vi "FIFO_AUTO_TEST.vi"() -> ()   [LabVIEW 2023]
uses:
  <vilib>/numeric/Random Number (Range) I64.vi
  deps/hdl-shared/host_interfaces/fifo/LabVIEW/HdlFifo/NiFpga_HdlFifo_WriteI64.vi
  deps/hdl-shared/host_interfaces/fifo/LabVIEW/HdlFifo/NiFpga_HdlFifo_ReadI64.vi
  <vilib>/numeric/Random Number (Range) DBL.vi
  deps/hdl-shared/host_interfaces/fifo/LabVIEW/HdlFifo/NiFpga_HdlFifo_WriteSGL.vi
  deps/hdl-shared/host_interfaces/fifo/LabVIEW/HdlFifo/NiFpga_HdlFifo_ReadSGL.vi
  <vilib>/numeric/Random Number (Range) U64.vi
  deps/hdl-shared/host_interfaces/fifo/LabVIEW/HdlFifo/NiFpga_HdlFifo_WriteU64.vi
  deps/hdl-shared/host_interfaces/fifo/LabVIEW/HdlFifo/NiFpga_HdlFifo_ReadU64.vi
  deps/hdl-shared/host_interfaces/fifo/LabVIEW/HdlFifo/NiFpga_HdlFifo_WriteBool.vi
  deps/hdl-shared/host_interfaces/fifo/LabVIEW/HdlFifo/NiFpga_HdlFifo_ReadBool.vi
  deps/hdl-shared/host_interfaces/fifo/LabVIEW/HdlFifo/NiFpga_HdlFifo_WriteI8.vi
  deps/hdl-shared/host_interfaces/fifo/LabVIEW/HdlFifo/NiFpga_HdlFifo_ReadI8.vi
  deps/hdl-shared/host_interfaces/fifo/LabVIEW/HdlFifo/NiFpga_HdlFifo_WriteU16.vi
  deps/hdl-shared/host_interfaces/fifo/LabVIEW/HdlFifo/NiFpga_HdlFifo_ReadU16.vi
  deps/hdl-shared/host_interfaces/fifo/LabVIEW/HdlFifo/NiFpga_HdlFifo_WriteI32.vi
  deps/hdl-shared/host_interfaces/fifo/LabVIEW/HdlFifo/NiFpga_HdlFifo_ReadI32.vi
  <vilib>/numeric/sub_Random U32.vi
  <vilib>/FPGAPlugInAG/Dynamic/niLvFpga_Download_Dynamic.vi
  <vilib>/FPGAPlugInAG/Dynamic/niLvFpga_Run_Dynamic.vi
  deps/hdl-shared/host_interfaces/fifo/LabVIEW/HdlFifo/NiFpga_HdlFifo_AddI64.vi
  deps/hdl-shared/host_interfaces/fifo/LabVIEW/HdlFifo/private/_NiFpga_HdlFifo_GetStream.vi
  <vilib>/Utility/error.llb/Error Cluster From Error Code.vi
  deps/hdl-shared/host_interfaces/fifo/LabVIEW/HdlFifo/NiFpga_HdlFifo_AddSGL.vi
  deps/hdl-shared/host_interfaces/fifo/LabVIEW/HdlFifo/NiFpga_HdlFifo_AddU64.vi
  deps/hdl-shared/host_interfaces/fifo/LabVIEW/HdlFifo/NiFpga_HdlFifo_AddBool.vi
  deps/hdl-shared/host_interfaces/fifo/LabVIEW/HdlFifo/NiFpga_HdlFifo_AddI8.vi
  deps/hdl-shared/host_interfaces/fifo/LabVIEW/HdlFifo/NiFpga_HdlFifo_AddU16.vi
  deps/hdl-shared/host_interfaces/fifo/LabVIEW/HdlFifo/NiFpga_HdlFifo_AddI32.vi
  <vilib>/rvi/interface/nirviMethod/nirviMethod.xnode
panel:
  in  "Access non-existant FIFOs":bool
  out "error out 8":errorcluster
  out "Non-Existant FIFO test status":bool
  in  "I64 Multiplier 2":sgl
  out "Numeric 9":i32
  in  "SGL Multiplier":dbl
  in  "U64 Multiplier":sgl
  in  "I8 Multiplier":sgl
  in  "U16 Multiplier":sgl
  in  "I32 Multiplier":sgl
  in  "I64 Multiplier":sgl
  out "error out 7":errorcluster
  out "I64 Pass":bool
  out "Numeric 8":i32
  out "WriteData 6":i64[](array[numeric])
  out "ReadData 6":i64[](array[numeric])
  in  "Device address":string="PXI1Slot2"
  in  "Bitfile path":path=path "C:/shared/github15-test/MacallanTop_GH15_7dmatest_3.lvbitx"
  out "data out":bool[](array[boolean])
  out "Array":bool[](array[boolean])
  out "Numeric 2":i32
  out "Boolean Pass":bool
  out "Numeric 7":i32
  out "WriteData 5":u64[](array[numeric])
  out "ReadData 5":u64[](array[numeric])
  out "U64 Pass":bool
  out "Numeric 6":i32
  out "WriteData 4":sgl[](array[numeric])
  out "ReadData 4":sgl[](array[numeric])
  out "SGL Pass":bool
  out "error out 6":errorcluster
  out "error out 5":errorcluster
  out "error out 4":errorcluster
  out "error out 3":errorcluster
  out "error out 2":errorcluster
  out "error out":errorcluster
  out "Numeric 5":i32
  out "WriteData 3":i8[](array[numeric])
  out "ReadData 3":i8[](array[numeric])
  out "I8 Pass":bool
  out "Numeric 4":i32
  out "WriteData 2":u16[](array[numeric])
  out "ReadData 2":u16[](array[numeric])
  out "U16 Pass":bool
  out "ReadData":i32[](array[numeric])
  out "WriteData":i32[](array[numeric])
  out "Numeric":i32
  out "I32 Pass":bool
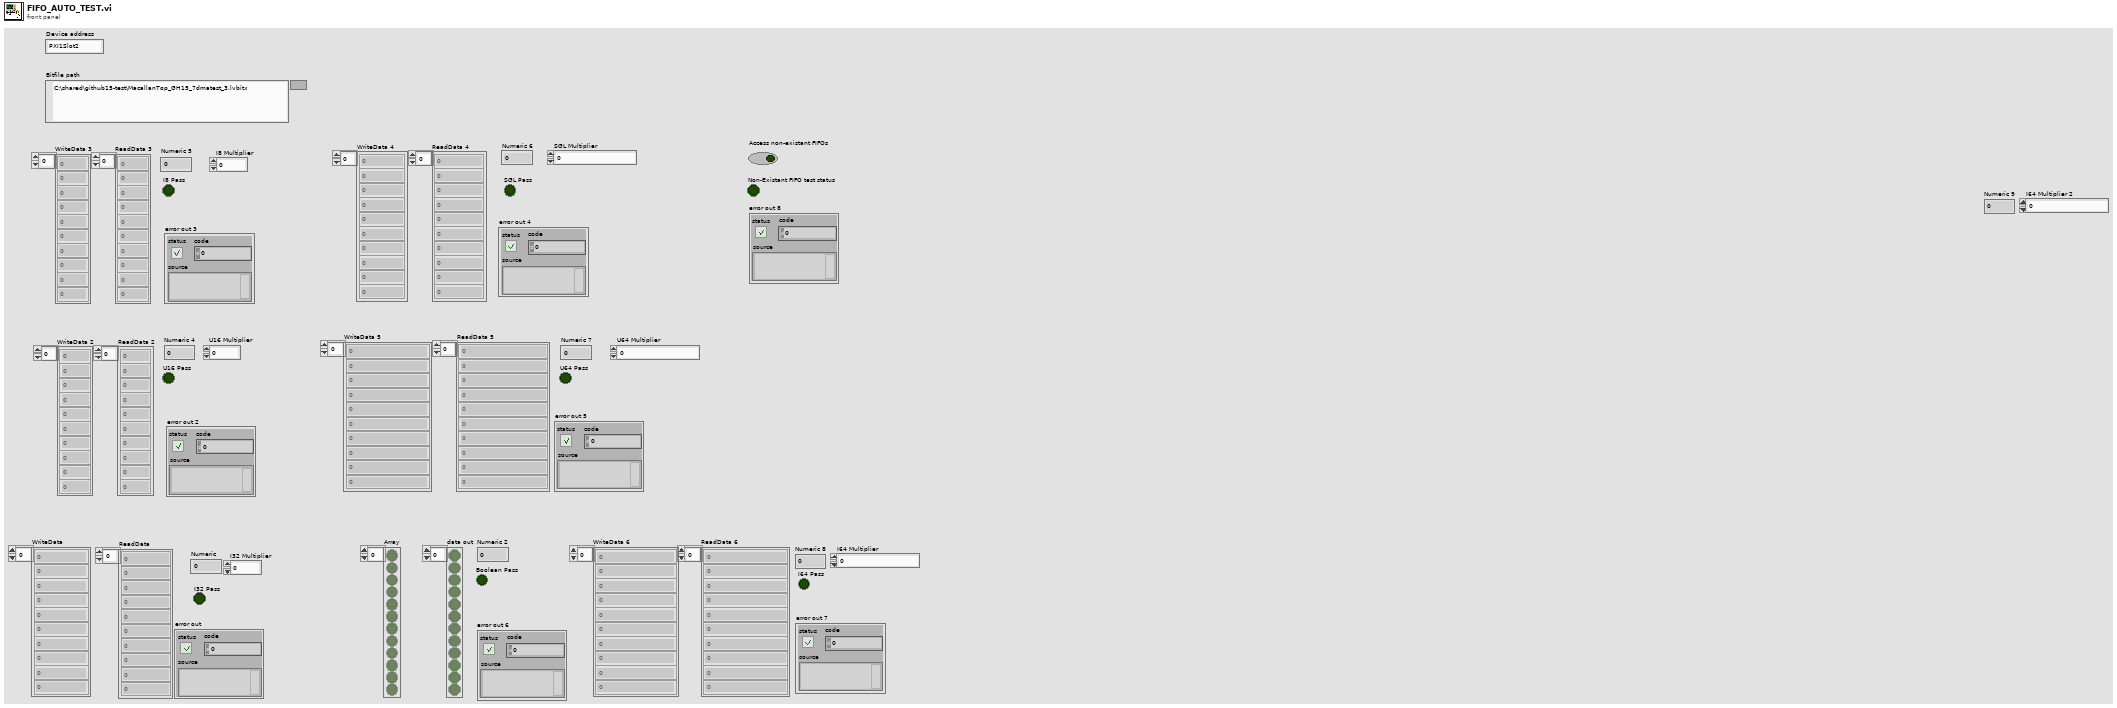
[diagram p1: front panel]
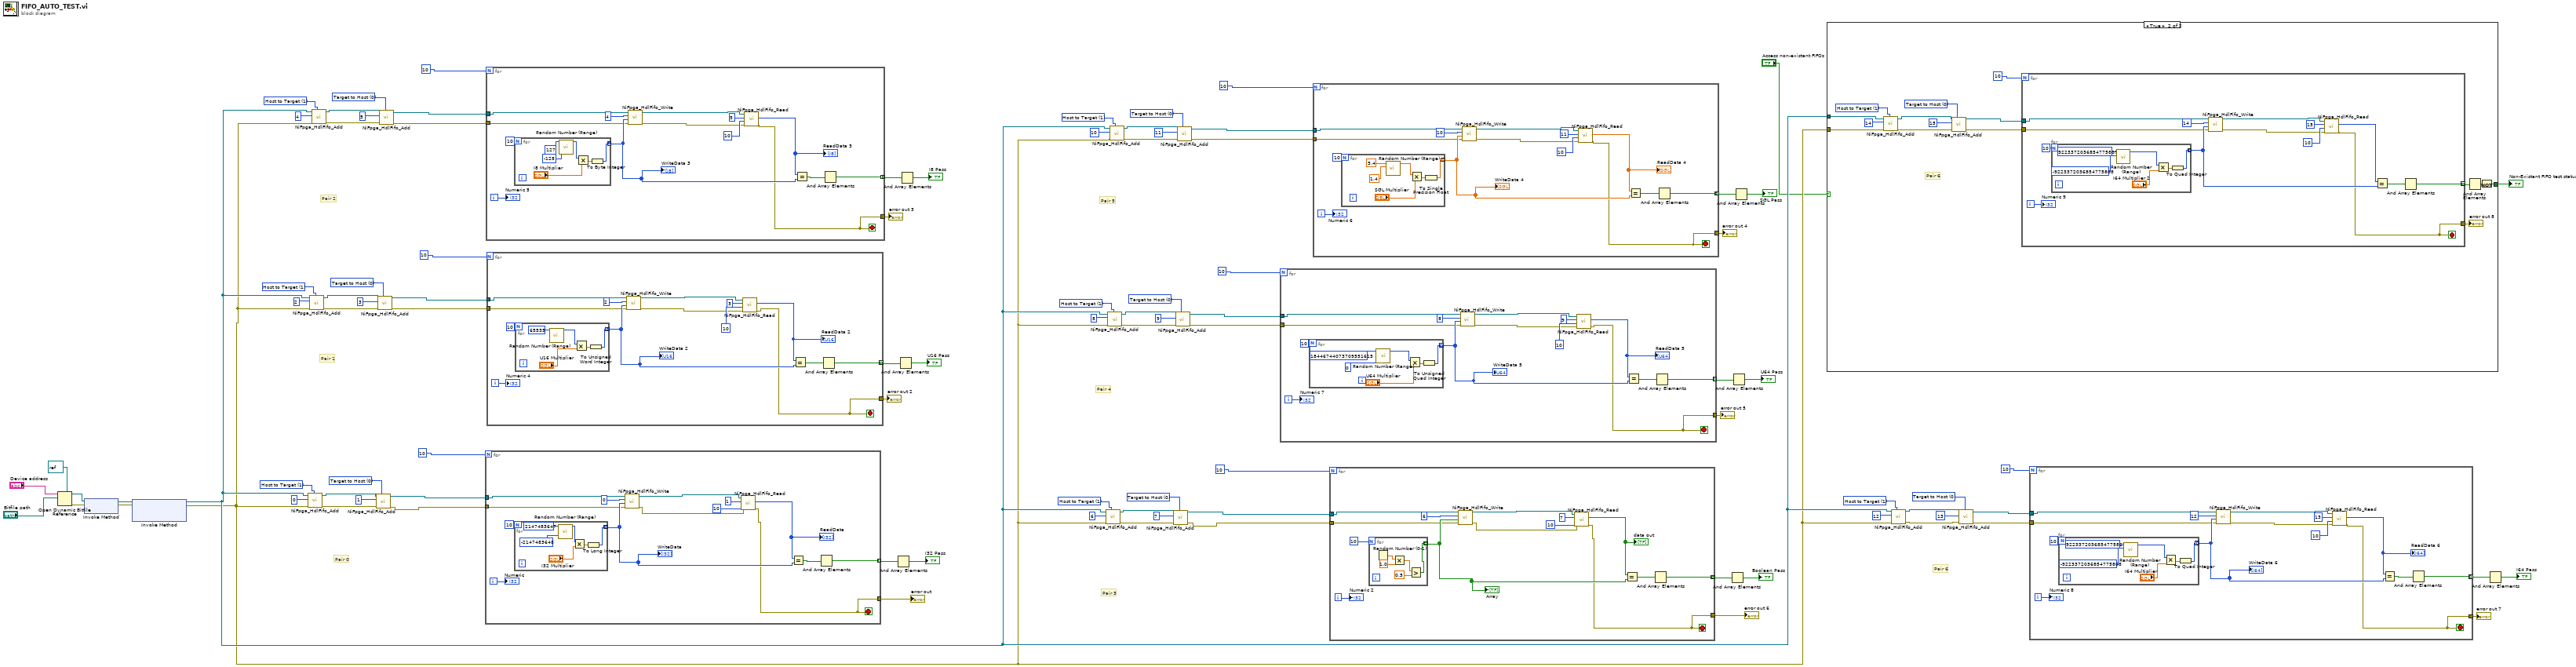
[diagram p0: block diagram]
diagram:
  w10 = u32 0 items=["Target to Host", "Host to Target"] ("direction")
  w6 = u32 1 items=["Target to Host", "Host to Target"]
  w39 = u32 0 items=["Target to Host", "Host to Target"] ("direction")
  w35 = u32 1 items=["Target to Host", "Host to Target"]
  w30 = u32 0 items=["Target to Host", "Host to Target"] ("direction")
  w34 = u32 1 items=["Target to Host", "Host to Target"]
  w21 = u32 0 items=["Target to Host", "Host to Target"] ("direction")
  w17 = u32 1 items=["Target to Host", "Host to Target"]
  w66 = u32 0 items=["Target to Host", "Host to Target"] ("direction")
  w70 = u32 1 items=["Target to Host", "Host to Target"]
  w75 = u32 0 items=["Target to Host", "Host to Target"] ("direction")
  w71 = u32 1 items=["Target to Host", "Host to Target"]
  w85 = u32 0 items=["Target to Host", "Host to Target"] ("direction")
  w89 = u32 1 items=["Target to Host", "Host to Target"]
  # "Pair 6"
  # "Pair 5"
  # "Pair 4"
  # "Pair 3"
  # "Pair 2"
  # "Pair 1"
  # "Pair 0"
  n1 = Open Dynamic Bitfile Reference(0:"Device address", 1:"Bitfile path", 4:refnum<k20> refnum ("Type")) -> (5:w92:refnum<k20>, 8:w91:errorcluster)  [unwired: 2 in]
  n2 = xnode "Invoke Method"("FPGA VI Reference In"=w92, "error in"=w91) -> ("FPGA VI Reference Out"=w94:refnum<k20>, "error out"=w95:errorcluster)
  n3 = xnode "Invoke Method"("FPGA VI Reference In"=w94, "error in"=w95) -> ("FPGA VI Reference Out"=w3:refnum<k20>, "error out"=w2:errorcluster)  [unwired: 1 in]
  n4 = call-poly "NiFpga_HdlFifo_Add.vi"("direction"=w89, "error in (no error)"=w2, "Fifo Number"=u32 0, "FPGA VI Reference In"=w3) -> ("error out"=w83:errorcluster, "FPGA VI Reference Out"=w87:refnum<k20>)  [unwired: 6 in]
  n5 = call-poly "NiFpga_HdlFifo_Add.vi"("direction"=w71, "error in (no error)"=w2, "Fifo Number"=u32 2, "FPGA VI Reference In"=w3) -> ("error out"=w76:errorcluster, "FPGA VI Reference Out"=w73:refnum<k20>)  [unwired: 6 in]
  n6 = call-poly "NiFpga_HdlFifo_Add.vi"("direction"=w70, "error in (no error)"=w2, "Fifo Number"=u32 4, "FPGA VI Reference In"=w3) -> ("error out"=w65:errorcluster, "FPGA VI Reference Out"=w68:refnum<k20>)  [unwired: 6 in]
  n7 = call-poly "NiFpga_HdlFifo_Add.vi"("direction"=w85, "error in (no error)"=w83, "Fifo Number"=u32 1, "FPGA VI Reference In"=w87) -> ("error out"=w58:errorcluster, "FPGA VI Reference Out"=w60:refnum<k20>)  [unwired: 6 in]
  n8 = call-poly "NiFpga_HdlFifo_Add.vi"("direction"=w75, "error in (no error)"=w76, "Fifo Number"=u32 3, "FPGA VI Reference In"=w73) -> ("error out"=w56:errorcluster, "FPGA VI Reference Out"=w61:refnum<k20>)  [unwired: 6 in]
  n9 = call-poly "NiFpga_HdlFifo_Add.vi"("direction"=w66, "error in (no error)"=w65, "Fifo Number"=u32 5, "FPGA VI Reference In"=w68) -> ("error out"=w54:errorcluster, "FPGA VI Reference Out"=w59:refnum<k20>)  [unwired: 6 in]
  n10 = for {
    N: 10 -> [_]
    tunnel: w60 -> [w106]
    tunnel: [w105] -> w81 mode=indexing
    tunnel: w58 -> [w99]
    tunnel: [w97] -> w57
    i -> [w101]
    stop <- w97 stop-if-true
    n11 = for {
      N: 10 -> [_]
      tunnel: [w113] -> w102 mode=indexing
      n12 = call-poly <vilib>:"Random Number (Range).vi"("lower bound (-100)"=i64 -2147483648, "upper bound (100)"=i64 2147483647) -> ("number"=w115:i64)  [unwired: 9 in]
      n13 = Multiply(x=w115, y="I32 Multiplier") -> (x*y=w114:sgl)
      n14 = To Long Integer(number=w114) -> (32bit integer=w113:i32)
    }
    "WriteData" <- w102
    n15 = call-poly "NiFpga_HdlFifo_Write.vi"("error in (no error)"=w99, "data in"=w102, "fifo number"=u32 0 ("Fifo Number 2"), "fpga vi reference in"=w106) -> ("error out"=w98:errorcluster, "fpga vi reference out"=w96:refnum<k20>)  [unwired: 4 in, 1 out]
    n16 = call-poly "NiFpga_HdlFifo_Read.vi"("error in (no error)"=w98, "number of elements"=10, "fifo number"=u32 1 ("Fifo Number"), "fpga vi reference in"=w96) -> ("error out"=w97:errorcluster, "data out"=w103:i32[])  [unwired: 3 in, 2 out]
    "ReadData" <- w103
    n17 = Equal?(x=w103, y=w102) -> (x = y?=w104:bool[])
    n18 = And Array Elements(Boolean array=w104) -> (logical AND=w105:bool)
    "Numeric" <- w101
  }
  "error out" <- w57
  n19 = for {
    N: 10 -> [_]
    tunnel: w59 -> [w126]
    tunnel: [w125] -> w63 mode=indexing
    tunnel: w54 -> [w119]
    tunnel: [w116] -> w53
    i -> [w121]
    stop <- w116 stop-if-true
    n20 = for {
      N: 10 -> [_]
      tunnel: [w133] -> w122 mode=indexing
      n21 = call-poly <vilib>:"Random Number (Range).vi"("lower bound (-100)"=i64 -128, "upper bound (100)"=i64 127) -> ("number"=w135:i64)  [unwired: 9 in]
      n22 = Multiply(x=w135, y="I8 Multiplier") -> (x*y=w134:sgl)
      n23 = To Byte Integer(number=w134) -> (8bit integer=w133:i8)
    }
    "WriteData 3" <- w122
    n24 = call-poly "NiFpga_HdlFifo_Write.vi"("error in (no error)"=w119, "data in"=w122, "fifo number"=u32 4 ("Fifo Number 2"), "fpga vi reference in"=w126) -> ("error out"=w118:errorcluster, "fpga vi reference out"=w117:refnum<k20>)  [unwired: 4 in, 1 out]
    n25 = call-poly "NiFpga_HdlFifo_Read.vi"("error in (no error)"=w118, "number of elements"=10, "fifo number"=u32 5 ("Fifo Number"), "fpga vi reference in"=w117) -> ("error out"=w116:errorcluster, "data out"=w123:i8[])  [unwired: 3 in, 2 out]
    "ReadData 3" <- w123
    n26 = Equal?(x=w123, y=w122) -> (x = y?=w124:bool[])
    n27 = And Array Elements(Boolean array=w124) -> (logical AND=w125:bool)
    "Numeric 5" <- w121
  }
  "error out 3" <- w53
  n28 = for {
    N: 10 -> [_]
    tunnel: w61 -> [w146]
    tunnel: [w145] -> w78 mode=indexing
    tunnel: w56 -> [w139]
    tunnel: [w136] -> w55
    i -> [w141]
    stop <- w136 stop-if-true
    n29 = for {
      N: 10 -> [_]
      tunnel: [w152] -> w142 mode=indexing
      n30 = call-poly <vilib>:"Random Number (Range).vi"("upper bound (100)"=u64 65535) -> ("number"=w154:u64)  [unwired: 10 in]
      n31 = Multiply(x=w154, y="U16 Multiplier") -> (x*y=w153:sgl)
      n32 = To Unsigned Word Integer(number=w153) -> (unsigned 16bit integer=w152:u16)
    }
    "WriteData 2" <- w142
    n33 = call-poly "NiFpga_HdlFifo_Write.vi"("error in (no error)"=w139, "data in"=w142, "fifo number"=u32 2 ("Fifo Number 2"), "fpga vi reference in"=w146) -> ("error out"=w138:errorcluster, "fpga vi reference out"=w137:refnum<k20>)  [unwired: 4 in, 1 out]
    n34 = call-poly "NiFpga_HdlFifo_Read.vi"("error in (no error)"=w138, "number of elements"=10, "fifo number"=u32 3 ("Fifo Number"), "fpga vi reference in"=w137) -> ("error out"=w136:errorcluster, "data out"=w143:u16[])  [unwired: 3 in, 2 out]
    "ReadData 2" <- w143
    n35 = Equal?(x=w143, y=w142) -> (x = y?=w144:bool[])
    n36 = And Array Elements(Boolean array=w144) -> (logical AND=w145:bool)
    "Numeric 4" <- w141
  }
  "error out 2" <- w55
  n37 = And Array Elements(Boolean array=w81) -> (logical AND=→"I32 Pass":bool)
  n38 = And Array Elements(Boolean array=w78) -> (logical AND=→"U16 Pass":bool)
  n39 = And Array Elements(Boolean array=w63) -> (logical AND=→"I8 Pass":bool)
  n40 = call-poly "NiFpga_HdlFifo_Add.vi"("direction"=w17, "error in (no error)"=w2, "Fifo Number"=u32 6, "FPGA VI Reference In"=w3) -> ("error out"=w22:errorcluster, "FPGA VI Reference Out"=w19:refnum<k20>)  [unwired: 6 in]
  n41 = call-poly "NiFpga_HdlFifo_Add.vi"("direction"=w34, "error in (no error)"=w2, "Fifo Number"=u32 8, "FPGA VI Reference In"=w3) -> ("error out"=w29:errorcluster, "FPGA VI Reference Out"=w32:refnum<k20>)  [unwired: 6 in]
  n42 = call-poly "NiFpga_HdlFifo_Add.vi"("direction"=w35, "error in (no error)"=w2, "Fifo Number"=u32 10, "FPGA VI Reference In"=w3) -> ("error out"=w40:errorcluster, "FPGA VI Reference Out"=w37:refnum<k20>)  [unwired: 6 in]
  n43 = call-poly "NiFpga_HdlFifo_Add.vi"("direction"=w21, "error in (no error)"=w22, "Fifo Number"=u32 7, "FPGA VI Reference In"=w19) -> ("error out"=w47:errorcluster, "FPGA VI Reference Out"=w45:refnum<k20>)  [unwired: 6 in]
  n44 = call-poly "NiFpga_HdlFifo_Add.vi"("direction"=w30, "error in (no error)"=w29, "Fifo Number"=u32 9, "FPGA VI Reference In"=w32) -> ("error out"=w49:errorcluster, "FPGA VI Reference Out"=w44:refnum<k20>)  [unwired: 6 in]
  n45 = call-poly "NiFpga_HdlFifo_Add.vi"("direction"=w39, "error in (no error)"=w40, "Fifo Number"=u32 11, "FPGA VI Reference In"=w37) -> ("error out"=w51:errorcluster, "FPGA VI Reference Out"=w46:refnum<k20>)  [unwired: 6 in]
  n46 = for {
    N: 10 -> [_]
    tunnel: w44 -> [w165]
    tunnel: [w164] -> w27 mode=indexing
    tunnel: w49 -> [w158]
    tunnel: [w155] -> w50
    i -> [w160]
    stop <- w155 stop-if-true
    n47 = for {
      N: 10 -> [_]
      tunnel: [w172] -> w161 mode=indexing
      n48 = call-poly <vilib>:"Random Number (Range).vi"("lower bound (0)"=u64 0, "upper bound (100)"=u64 18446744073709551615) -> ("number"=w174:u64)  [unwired: 9 in]
      n49 = Multiply(x=w174, y="U64 Multiplier") -> (x*y=w173:sgl)
      n50 = To Unsigned Quad Integer(1:w173) -> (0:w172:u64)
    }
    "WriteData 5" <- w161
    n51 = call-poly "NiFpga_HdlFifo_Write.vi"("error in (no error)"=w158, "data in"=w161, "fifo number"=u32 8 ("Fifo Number 2"), "fpga vi reference in"=w165) -> ("error out"=w157:errorcluster, "fpga vi reference out"=w156:refnum<k20>)  [unwired: 4 in, 1 out]
    n52 = call-poly "NiFpga_HdlFifo_Read.vi"("error in (no error)"=w157, "number of elements"=10, "fifo number"=u32 9 ("Fifo Number"), "fpga vi reference in"=w156) -> ("error out"=w155:errorcluster, "data out"=w162:u64[])  [unwired: 3 in, 2 out]
    "ReadData 5" <- w162
    n53 = Equal?(x=w162, y=w161) -> (x = y?=w163:bool[])
    n54 = And Array Elements(Boolean array=w163) -> (logical AND=w164:bool)
    "Numeric 7" <- w160
  }
  "error out 5" <- w50
  n55 = for {
    N: 10 -> [_]
    tunnel: w46 -> [w185]
    tunnel: [w184] -> w42 mode=indexing
    tunnel: w51 -> [w178]
    tunnel: [w175] -> w52
    i -> [w180]
    stop <- w175 stop-if-true
    n56 = for {
      N: 10 -> [_]
      tunnel: [w192] -> w181 mode=indexing
      n57 = call-poly <vilib>:"Random Number (Range).vi"("lower bound (0)"=1.4 ("lower bound (-100)"), "upper bound (100)"=3.4) -> ("number"=w194:dbl)  [unwired: 9 in]
      n58 = Multiply(x=w194, y="SGL Multiplier") -> (x*y=w193:dbl)
      n59 = To Single Precision Float(number=w193) -> (single precision float=w192:sgl)
    }
    "WriteData 4" <- w181
    n60 = call-poly "NiFpga_HdlFifo_Write.vi"("error in (no error)"=w178, "data in"=w181, "fifo number"=u32 10 ("Fifo Number 2"), "fpga vi reference in"=w185) -> ("error out"=w177:errorcluster, "fpga vi reference out"=w176:refnum<k20>)  [unwired: 4 in, 1 out]
    n61 = call-poly "NiFpga_HdlFifo_Read.vi"("error in (no error)"=w177, "number of elements"=10, "fifo number"=u32 11 ("Fifo Number"), "fpga vi reference in"=w176) -> ("error out"=w175:errorcluster, "data out"=w182:sgl[])  [unwired: 3 in, 2 out]
    "ReadData 4" <- w182
    n62 = Equal?(x=w182, y=w181) -> (x = y?=w183:bool[])
    n63 = And Array Elements(Boolean array=w183) -> (logical AND=w184:bool)
    "Numeric 6" <- w180
  }
  "error out 4" <- w52
  n64 = for {
    N: 10 -> [_]
    tunnel: w45 -> [w205]
    tunnel: [w204] -> w24 mode=indexing
    tunnel: w47 -> [w198]
    tunnel: [w196] -> w48
    i -> [w200]
    stop <- w196 stop-if-true
    n65 = for {
      N: 10 -> [_]
      tunnel: [w209] -> w201 mode=indexing
      n66 = Random Number (0-1)() -> (number: 0 to 1=w213:dbl)
      n67 = Multiply(x=w213, y=1.0) -> (x*y=w211:dbl)
      n68 = Greater?(x=w211, y=0.5) -> (0:w209:bool)
    }
    "Array" <- w201
    n69 = call-poly "NiFpga_HdlFifo_Write.vi"("error in (no error)"=w198, "data in"=w201, "fifo number"=u32 6 ("Fifo Number 2"), "fpga vi reference in"=w205) -> ("error out"=w197:errorcluster, "fpga vi reference out"=w195:refnum<k20>)  [unwired: 4 in, 1 out]
    n70 = call-poly "NiFpga_HdlFifo_Read.vi"("error in (no error)"=w197, "number of elements"=10, "fifo number"=u32 7 ("Fifo Number"), "fpga vi reference in"=w195) -> ("error out"=w196:errorcluster, "data out"=w202:bool[])  [unwired: 3 in, 2 out]
    "data out" <- w202
    n71 = Equal?(x=w202, y=w201) -> (x = y?=w203:bool[])
    n72 = And Array Elements(Boolean array=w203) -> (logical AND=w204:bool)
    "Numeric 2" <- w200
  }
  "error out 6" <- w48
  n73 = And Array Elements(Boolean array=w24) -> (logical AND=→"Boolean Pass":bool)
  n74 = And Array Elements(Boolean array=w27) -> (logical AND=→"U64 Pass":bool)
  n75 = And Array Elements(Boolean array=w42) -> (logical AND=→"SGL Pass":bool)
  n76 = case shown="True" "Access non-existant FIFOs" {
    selector: "Access non-existant FIFOs" -> [w214 _]
    tunnel: [w214 w216] -> w4
    tunnel: w3 -> [_ w229]
    tunnel: w2 -> [_ w228]
    frame False {
    }
    frame True {
      w222 = u32 0 items=["Target to Host", "Host to Target"] ("direction")
      w218 = u32 1 items=["Target to Host", "Host to Target"]
      # "Pair 6"
      n77 = call-poly "NiFpga_HdlFifo_Add.vi"("direction"=w218, "error in (no error)"=w228, "Fifo Number"=u32 14, "FPGA VI Reference In"=w229) -> ("error out"=w223:errorcluster, "FPGA VI Reference Out"=w220:refnum<k20>)  [unwired: 6 in]
      n78 = call-poly "NiFpga_HdlFifo_Add.vi"("direction"=w222, "error in (no error)"=w223, "Fifo Number"=u32 15, "FPGA VI Reference In"=w220) -> ("error out"=w217:errorcluster, "FPGA VI Reference Out"=w226:refnum<k20>)  [unwired: 6 in]
      n79 = for {
        N: 10 -> [_]
        tunnel: w226 -> [w240]
        tunnel: [w239] -> w225 mode=indexing
        tunnel: w217 -> [w233]
        tunnel: [w230] -> w227
        i -> [w235]
        stop <- w230 stop-if-true
        n80 = for {
          N: 10 -> [_]
          tunnel: [w247] -> w236 mode=indexing
          n81 = call-poly <vilib>:"Random Number (Range).vi"("lower bound (-100)"=i64 -9223372036854775808, "upper bound (100)"=i64 9223372036854775807) -> ("number"=w249:i64)  [unwired: 9 in]
          n82 = Multiply(x=w249, y="I64 Multiplier 2") -> (x*y=w248:sgl)
          n83 = To Quad Integer(1:w248) -> (0:w247:i64)
        }
        n84 = call-poly "NiFpga_HdlFifo_Write.vi"("error in (no error)"=w233, "data in"=w236, "fifo number"=u32 14 ("Fifo Number 2"), "fpga vi reference in"=w240) -> ("error out"=w232:errorcluster, "fpga vi reference out"=w231:refnum<k20>)  [unwired: 4 in, 1 out]
        n85 = call-poly "NiFpga_HdlFifo_Read.vi"("error in (no error)"=w232, "number of elements"=10, "fifo number"=u32 15 ("Fifo Number"), "fpga vi reference in"=w231) -> ("error out"=w230:errorcluster, "data out"=w237:i64[])  [unwired: 3 in, 2 out]
        n86 = Equal?(x=w237, y=w236) -> (x = y?=w238:bool[])
        n87 = And Array Elements(Boolean array=w238) -> (logical AND=w239:bool)
        "Numeric 9" <- w235
      }
      "error out 8" <- w227
      n88 = And Array Elements(Boolean array=w225) -> (logical AND=w215:bool)
      n89 = Not(x=w215) -> (.not. x?=w216:bool)
    }
  }
  "Non-Existant FIFO test status" <- w4
  n90 = call-poly "NiFpga_HdlFifo_Add.vi"("direction"=w6, "error in (no error)"=w2, "Fifo Number"=u32 12, "FPGA VI Reference In"=w3) -> ("error out"=w11:errorcluster, "FPGA VI Reference Out"=w8:refnum<k20>)  [unwired: 6 in]
  n91 = call-poly "NiFpga_HdlFifo_Add.vi"("direction"=w10, "error in (no error)"=w11, "Fifo Number"=u32 13, "FPGA VI Reference In"=w8) -> ("error out"=w5:errorcluster, "FPGA VI Reference Out"=w15:refnum<k20>)  [unwired: 6 in]
  n92 = for {
    N: 10 -> [_]
    tunnel: w15 -> [w260]
    tunnel: [w259] -> w13 mode=indexing
    tunnel: w5 -> [w253]
    tunnel: [w250] -> w16
    i -> [w255]
    stop <- w250 stop-if-true
    n93 = for {
      N: 10 -> [_]
      tunnel: [w267] -> w256 mode=indexing
      n94 = call-poly <vilib>:"Random Number (Range).vi"("lower bound (-100)"=i64 -9223372036854775808, "upper bound (100)"=i64 9223372036854775807) -> ("number"=w269:i64)  [unwired: 9 in]
      n95 = Multiply(x=w269, y="I64 Multiplier") -> (x*y=w268:sgl)
      n96 = To Quad Integer(1:w268) -> (0:w267:i64)
    }
    "WriteData 6" <- w256
    n97 = call-poly "NiFpga_HdlFifo_Write.vi"("error in (no error)"=w253, "data in"=w256, "fifo number"=u32 12 ("Fifo Number 2"), "fpga vi reference in"=w260) -> ("error out"=w252:errorcluster, "fpga vi reference out"=w251:refnum<k20>)  [unwired: 4 in, 1 out]
    n98 = call-poly "NiFpga_HdlFifo_Read.vi"("error in (no error)"=w252, "number of elements"=10, "fifo number"=u32 13 ("Fifo Number"), "fpga vi reference in"=w251) -> ("error out"=w250:errorcluster, "data out"=w257:i64[])  [unwired: 3 in, 2 out]
    "ReadData 6" <- w257
    n99 = Equal?(x=w257, y=w256) -> (x = y?=w258:bool[])
    n100 = And Array Elements(Boolean array=w258) -> (logical AND=w259:bool)
    "Numeric 8" <- w255
  }
  "error out 7" <- w16
  n101 = And Array Elements(Boolean array=w13) -> (logical AND=→"I64 Pass":bool)
